vi "题4.2.vi"() -> ()   [LabVIEW 2017]
panel:
  in  "Digital Waveform":digitalwaveform(waveform)={"t0"=timestamp(0 s since 1904-01-01), "dt"=1.0, "Y"={"transitions"=[], "data"=[]}} caption="数字波形"
  out "数字波形图":digitalwaveform(graph)
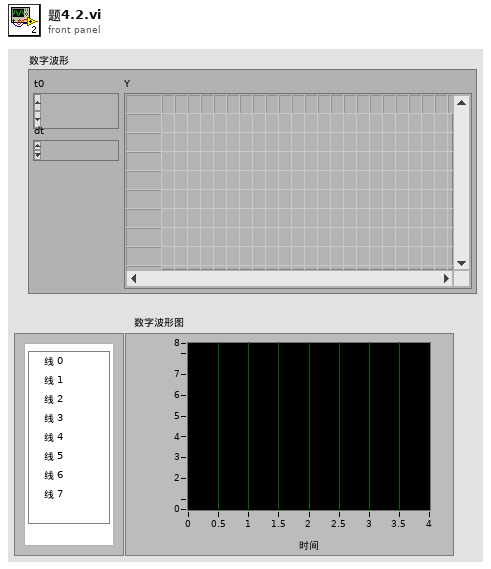
[diagram p1: front panel]
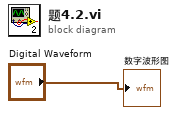
[diagram p0: block diagram]
diagram:
  "数字波形图" <- "Digital Waveform"
